vi "RI DFI Operation.vi"(8 "error in (no error)":errorcluster, 9 "DFI Source (0:Off)":u16(ring) items=["Off", "QUES", "OPER", "ESB", "RQS"], 10 "RI Mode (0:Off)":u16(ring) items=["Off", "Latching", "Live"], 11 "VISA resource name":refnum<visa-resource-name>) -> (0 "error out":errorcluster, 3 "VISA resource name out":refnum<visa-resource-name>)   [LabVIEW 2021, in "Keithley 2200 Series.lvlib"]
doc: "Configure the power supply for RI/DFI mode.\nRemote Inhibit:Inhibit Input controls the output state of the power supply.\nDiscrete Fault Interrupt - Output :The Fault Output can indicate the reason for internal failure."
uses:
  <instrlib>/Keithley 2200 Series/Keithley 2200 Series.lvlib
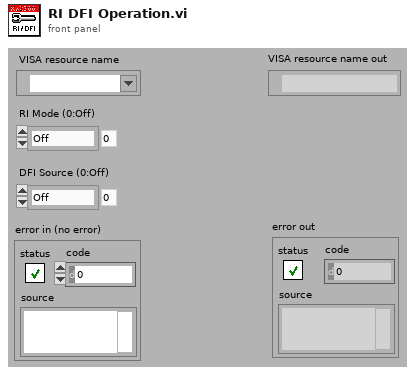
[diagram p1: front panel]
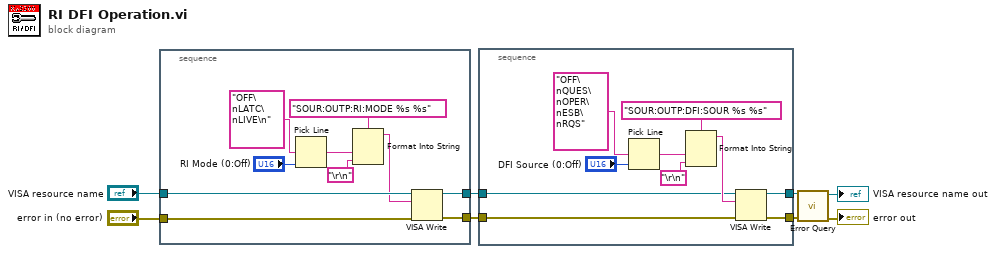
[diagram p0: block diagram]
diagram:
  n1 = stacked-sequence {
    tunnel: "VISA resource name" -> [w18]
    tunnel: "error in (no error)" -> [w17]
    tunnel: [w10] -> w4
    tunnel: [w9] -> w3
    frame #0 {
      n2 = Pick Line(multi-line string="OFF\nLATC\nLIVE\n" ("string (\"\")"), line index="RI Mode (0:Off)") -> (output string=w14:string)  [unwired: 1 out]
      n3 = Format Into String(format string="SOUR:OUTP:RI:MODE %s %s", w14, "\r\n" ("End of Line Constant")) -> (resulting string=w11:string)  [unwired: 2 in, 1 out]
      n4 = VISA Write(VISA resource name=w18, write buffer=w11, error in (no error)=w17) -> (VISA resource name out=w10:refnum<visa-resource-name>, error out=w9:errorcluster)  [unwired: 1 out]
    }
  }
  n5 = stacked-sequence {
    tunnel: w4 -> [w22]
    tunnel: w3 -> [w21]
    tunnel: [w20] -> w2
    tunnel: [w19] -> w1
    frame #0 {
      n6 = Pick Line(multi-line string="OFF\nQUES\nOPER\nESB\nRQS" ("string (\"\")"), line index="DFI Source (0:Off)") -> (output string=w27:string)  [unwired: 1 out]
      n7 = Format Into String(format string="SOUR:OUTP:DFI:SOUR %s %s", w27, "\r\n" ("End of Line Constant")) -> (resulting string=w23:string)  [unwired: 2 in, 1 out]
      n8 = VISA Write(VISA resource name=w22, write buffer=w23, error in (no error)=w21) -> (VISA resource name out=w20:refnum<visa-resource-name>, error out=w19:errorcluster)  [unwired: 1 out]
    }
  }
  n9 = call <instrlib>:"Error Query.vi"("error in (no error)"=w1, "VISA resource name"=w2) -> ("error out"=→"error out":errorcluster, "VISA resource name out"=→"VISA resource name out":refnum<visa-resource-name>)  [unwired: 8 out]
